vi "draw complex lorentzian.vi"(11 "4 corners":T1={"z (-pi/2)"=-1.0311345636926572+0.5736824521422934i, "z(inf)"=-0.5200164984937075+1.0975277942502903i, "z (pi/2)"=-1.0311345636926572+0.5736824521422934i, "z center"=-0.5136528600391839+0.580046090596817i, "z(0)"=-0.5200164984937075+1.0975277942502903i, "radius"=-1.0311345636926572}) -> (2 "fancy circles":cluster{dbl[], dbl[]}[](array[cluster]))   [LabVIEW 2017]
uses:
  circle corners.ctl
  generate linear region.vi
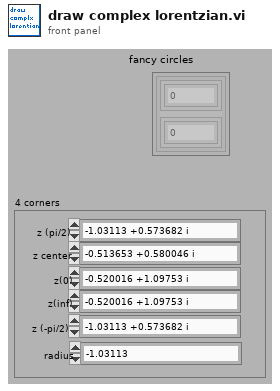
[diagram p1: front panel]
types:
  T1 = typedef "circle corners.ctl" = cluster{"z (-pi/2)":cdb, "z(inf)":cdb, "z (pi/2)":cdb, "z center":cdb, "z(0)":cdb, "radius":dbl}
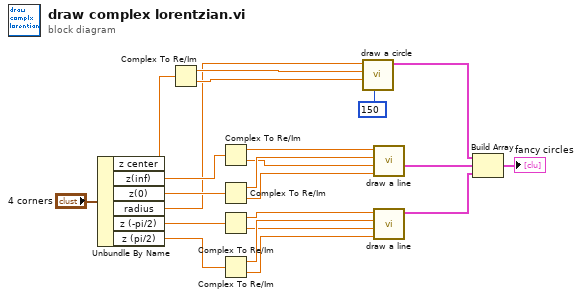
[diagram p0: block diagram]
diagram:
  n1 = Unbundle By Name("4 corners") -> ("z center"=w5:cdb, "z(inf)"=w3:cdb, "z(0)"=w4:cdb, "radius"=w2:dbl, "z (-pi/2)"=w11:cdb, "z (pi/2)"=w10:cdb)
  n2 = Complex To Re/Im(x + iy=w5) -> (x=w16:dbl, y=w17:dbl)
  n3 = Complex To Re/Im(x + iy=w3) -> (x=w21:dbl, y=w19:dbl)
  n4 = Complex To Re/Im(x + iy=w4) -> (x=w20:dbl, y=w18:dbl)
  n5 = Complex To Re/Im(x + iy=w11) -> (x=w15:dbl, y=w13:dbl)
  n6 = Complex To Re/Im(x + iy=w10) -> (x=w14:dbl, y=w12:dbl)
  n7 = call "draw a circle.vi"("number of points"=150, "center Y"=w17, "center x"=w16, "radius"=w2) -> ("output cluster"=w22:cluster{dbl[], dbl[]})  [unwired: 7 in]
  n8 = call "draw a line.vi"("y1"=w18, "y0"=w19, "x1"=w20, "x0"=w21) -> ("output cluster"=w9:cluster{dbl[], dbl[]})  [unwired: 7 in]
  n9 = call "draw a line.vi"("y1"=w12, "y0"=w13, "x1"=w14, "x0"=w15) -> ("output cluster"=w8:cluster{dbl[], dbl[]})  [unwired: 7 in]
  n10 = Build Array(w22, w9, w8) -> (→"fancy circles":cluster{dbl[], dbl[]}[])
